vi "正弦分布指示灯（8）.vi"() -> ()   [LabVIEW 2011]
uses:
  <vilib>/Utility/miscctls.llb/LVBoundsTypeDef.ctl
  <vilib>/Analysis/NI_AALBase.lvlib
panel:
  in  "X间距":i32=20
  in  "amplitude":dbl=40.0 caption="幅值" format="%0.2f"
  in  "按钮大小":T1={"Width"=12, "Height"=12}
  out "Led7":bool=TRUE
  out "Led6":bool
  out "Led5":bool=TRUE
  out "Led4":bool
  out "Led3":bool
  out "Led2":bool
  out "Led1":bool
  out "Led0":bool
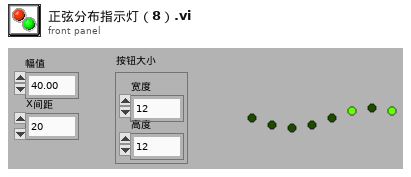
[diagram p1: front panel]
types:
  T1 = typedef "LVBoundsTypeDef.ctl" = cluster{"Width":u32, "Height":u32}
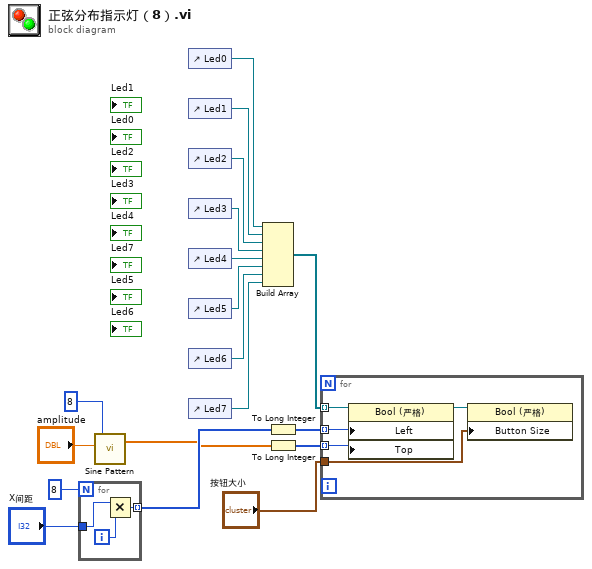
[diagram p0: block diagram]
diagram:
  n1 = for {
    N: 8 -> [_]
    tunnel: "X间距" -> [w20]
    tunnel: [w19] -> w2 mode=indexing
    i -> [w21]
    n2 = Multiply(x=w20, y=w21) -> (x*y=w19:i32)
  }
  n3 = call <vilib>:"Sine Pattern.vi"("amplitude"="amplitude", "samples"=8) -> ("Sinusoidal Pattern"=w1:dbl[])  [unwired: 2 in, 1 out]
  n4 = control-ref of="Led0"() -> (w18:refnum<vi>)
  n5 = control-ref of="Led1"() -> (w17:refnum<vi>)
  n6 = control-ref of="Led2"() -> (w16:refnum<vi>)
  n7 = control-ref of="Led3"() -> (w15:refnum<vi>)
  n8 = control-ref of="Led4"() -> (w14:refnum<vi>)
  n9 = control-ref of="Led5"() -> (w13:refnum<vi>)
  n10 = control-ref of="Led6"() -> (w12:refnum<vi>)
  n11 = control-ref of="Led7"() -> (w11:refnum<vi>)
  n12 = Build Array(w18, w17, w16, w15, w14, w13, w12, w11) -> (w10:refnum<vi>[])
  n13 = To Long Integer(number=w2) -> (32bit integer=w9:i32[])
  n14 = To Long Integer(number=w1) -> (32bit integer=w8:i32[])
  n15 = for {
    tunnel: w10 -> [w26] mode=indexing
    tunnel: w9 -> [w25] mode=indexing
    tunnel: w8 -> [w24] mode=indexing
    tunnel: "按钮大小" -> [w22]
    n16 = property class="Bool (严格)"(reference=w26, "Left"=w25, "Top"=w24) -> (reference out=w23:refnum<vi>)  [unwired: 1 in, 1 out]
    n17 = property class="Bool (严格)"(reference=w23, "Button Size"=w22) -> ()  [unwired: 1 in, 2 out]
  }
